vi "IndexFlowmeter.vi"() -> ()   [LabVIEW 2012]
panel:
  in  "IndexFlowmeter":cluster{"IndexFlowmeter":i32, "SwitchDelay":u16}
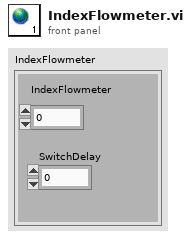
[diagram p1: front panel]
diagram:
